vi "Configure Offset and Limits (Adjacent Channel Power - Relative and Absolute Limits.vi"(0 "VISA resource name":refnum<visa-resource-name>, 1 "Relative Limit of PSD List":dbl[](array[numeric])=[-28.87, -28.87, -28.87, -28.87, -28.87, -28.87], 5 "Device Mode (1: BTS)":i32(ring)=1 items=["BTS"=1, "MS"=2], 7 "Fail Conditions List":i32[](array[ring])=[3, 3, 3, 3, 3, 3] items=["Absolute", "AND", "OR", "Relative"], 9 "Relative Limit of Carrier Level List":dbl[](array[numeric])=[-45.0, -45.0, -45.0, -45.0, -45.0, -45.0], 11 "error in (no error)":errorcluster, 12 "Absolute Limit List":dbl[](array[numeric])=[0.0, 0.0, 0.0, 0.0, 0.0, 0.0]) -> (4 "VISA resource name out":refnum<visa-resource-name>, 15 "error out":errorcluster)   [LabVIEW 2018, in "Agilent MXA Series.lvlib"]
doc: "Configures the absolute and relative limits settings under the offsets and limits for ACP measurement type."
uses:
  Agilent MXA Series.lvlib
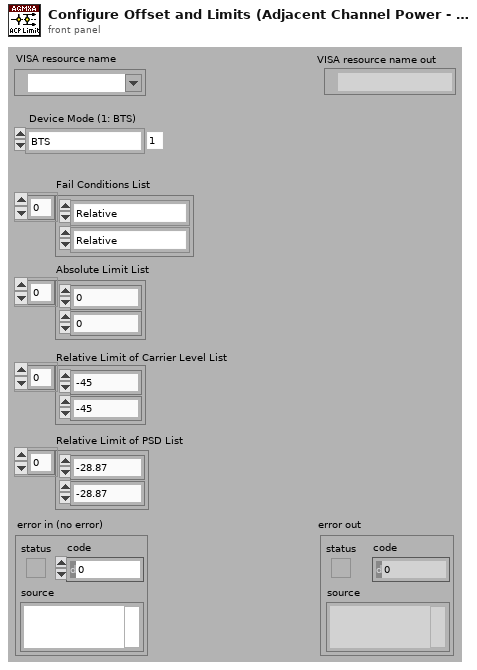
[diagram p1: front panel]
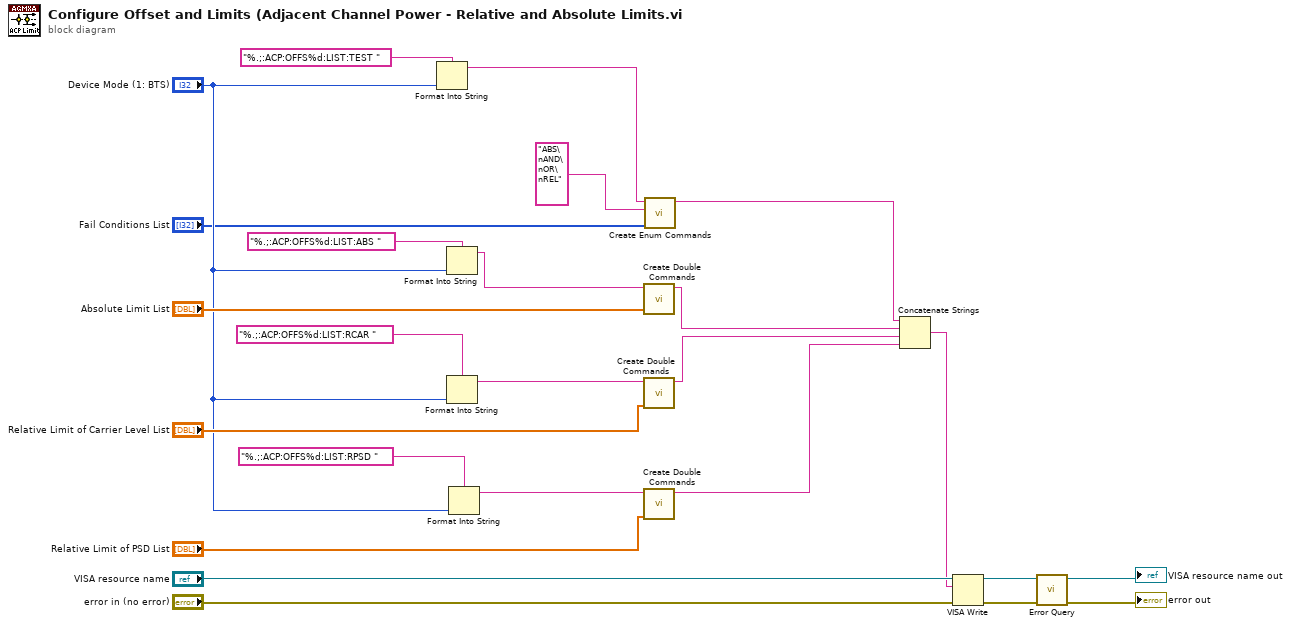
[diagram p0: block diagram]
diagram:
  n1 = Format Into String(format string="%.;:ACP:OFFS%d:LIST:TEST ", "Device Mode (1: BTS)") -> (resulting string=w2:string)  [unwired: 2 in, 1 out]
  n2 = Format Into String(format string="%.;:ACP:OFFS%d:LIST:ABS ", "Device Mode (1: BTS)") -> (resulting string=w23:string)  [unwired: 2 in, 1 out]
  n3 = Format Into String(format string="%.;:ACP:OFFS%d:LIST:RCAR ", "Device Mode (1: BTS)") -> (resulting string=w20:string)  [unwired: 2 in, 1 out]
  n4 = Format Into String(format string="%.;:ACP:OFFS%d:LIST:RPSD ", "Device Mode (1: BTS)") -> (resulting string=w16:string)  [unwired: 2 in, 1 out]
  n5 = call "Create Double Commands.vi"("Double Values"="Absolute Limit List", "Commands"=w23) -> ("Result"=w14:string)  [unwired: 9 in]
  n6 = call "Create Double Commands.vi"("Double Values"="Relative Limit of Carrier Level List", "Commands"=w20) -> ("Result"=w13:string)  [unwired: 9 in]
  n7 = call "Create Double Commands.vi"("Double Values"="Relative Limit of PSD List", "Commands"=w16) -> ("Result"=w12:string)  [unwired: 9 in]
  n8 = call "Create Enum Commands.vi"("Enum Values"="Fail Conditions List", "Multi-line Text"="ABS\nAND\nOR\nREL" ("multi-line string"), "Commands"=w2) -> ("Result"=w1:string)  [unwired: 8 in]
  n9 = Concatenate Strings(w1, w14, w13, w12) -> (w5:string)
  n10 = VISA Write(VISA resource name="VISA resource name", write buffer=w5, error in (no error)="error in (no error)") -> (VISA resource name out=w9:refnum<visa-resource-name>, error out=w8:errorcluster)  [unwired: 1 out]
  n11 = call "Error Query.vi"("error in (no error)"=w8, "VISA resource name"=w9) -> ("error out"=→"error out":errorcluster, "VISA resource name out"=→"VISA resource name out":refnum<visa-resource-name>)  [unwired: 6 in, 2 out]
